vi "Should Show Spectrogram Window.vi"(11 "Data in":T1={"First Time"=FALSE, "Show Spectrogram Window"=TRUE, "Show Spectrogram Window Button Clicked"=FALSE, "Extension"=0, "Time steps"=-1, "Frequency bins"=512, "Type"=1, "Length"=-1, "Color Table"=0, "Spectrogram VI Ref"=refnum} {"Color Table" items=["Rainbow", "Inverse gray", "Gray", "Color table 1", "Color table 2", "Color table 3"]; "Type" items=["None ", "Hanning", "Hamming", "Blackman-Harris", "Exact Blackman", "Blackman", "Flat Top", "4 Term B-Harris ", "7 Term B-Harris", "Low Sidelobe", "Gaussian"]; "Extension" items=["Zero padding", "Symmetric", "Periodic"]}) -> (2 "Show Window":bool, 3 "Data out":T1={"First Time"=FALSE, "Show Spectrogram Window"=TRUE, "Show Spectrogram Window Button Clicked"=FALSE, "Extension"=0, "Time steps"=-1, "Frequency bins"=512, "Type"=1, "Length"=-1, "Color Table"=0, "Spectrogram VI Ref"=refnum} {"Color Table" items=["Rainbow", "Inverse gray", "Gray", "Color table 1", "Color table 2", "Color table 3"]; "Type" items=["None ", "Hanning", "Hamming", "Blackman-Harris", "Exact Blackman", "Blackman", "Flat Top", "4 Term B-Harris ", "7 Term B-Harris", "Low Sidelobe", "Gaussian"]; "Extension" items=["Zero padding", "Symmetric", "Periodic"]})   [LabVIEW 2023, in "Spectrogram.lvlib" / "Spectrogram.lvclass"]
uses:
  Spectrogram.lvclass
  Spectrogram Data.ctl
  Spectrogram.lvclass/Spectrogram.ctl
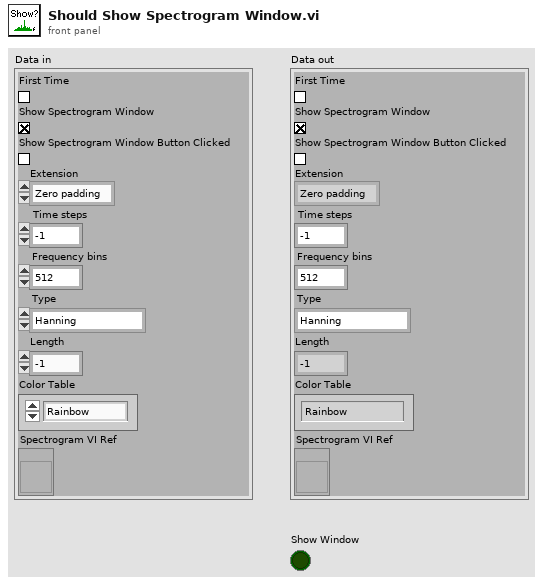
[diagram p1: front panel]
types:
  T1 = typedef "Spectrogram.lvlib/Spectrogram.lvclass/Spectrogram Data.ctl" = cluster{"First Time":bool, "Show Spectrogram Window":bool, "Show Spectrogram Window Button Clicked":bool, "Extension":u16, "Time steps":i32, "Frequency bins":i32, "Type":i32, "Length":i32, "Color Table":u16, "Spectrogram VI Ref":refnum<vi>}
  T2 = enum32{"Invalid", "Standard", "Closed", "Hidden", "Minimized", "Maximized"}
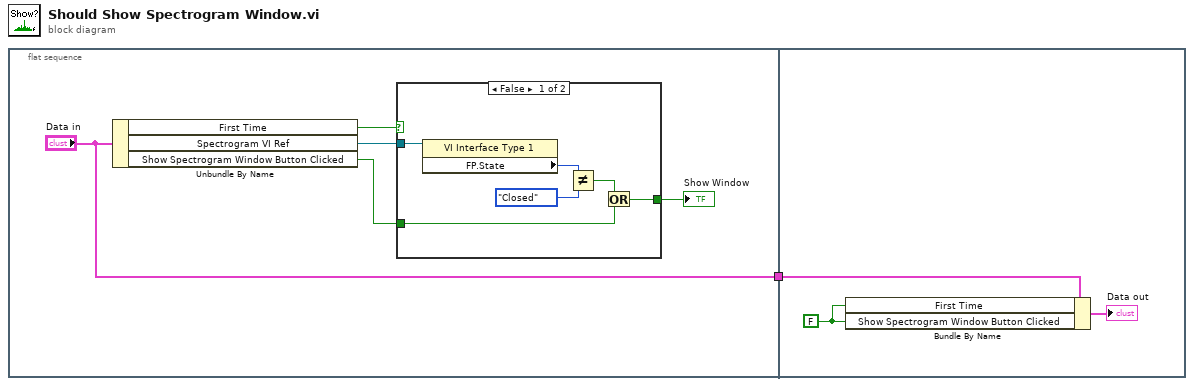
[diagram p0: block diagram]
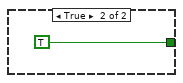
[diagram p2: hidden frame]
diagram:
  n1 = flat-sequence {
    tunnel: ["Data in"] -> w1
    tunnel: w1 -> [w16]
    frame #0 {
      n2 = Unbundle By Name("Data in") -> ("First Time"=w2:bool, "Spectrogram VI Ref"=w5:refnum<vi>, "Show Spectrogram Window Button Clicked"=w4:bool)
      n3 = case shown="False" w2 {
        tunnel: w5 -> [w12 _]
        tunnel: [w7 TRUE] -> w6
        tunnel: w4 -> [w9 _]
        frame False {
          n4 = property class="VI Interface Type 1"(reference=w12) -> ("FP.State"=w11:T2)  [unwired: 1 in, 2 out]
          n5 = Not Equal?(x=w11, y=T2."Closed" ("Front Panel Window:State")) -> (x != y?=w8:bool)
          n6 = Or(x=w8, y=w9) -> (x .or. y?=w7:bool)
        }
        frame True {
        }
      }
      "Show Window" <- w6
    }
    frame #1 {
      w14 = FALSE ("Show Spectrogram Window Button Clicked")
      n7 = Bundle By Name(cluster=w16, "First Time"=w14, "Show Spectrogram Window Button Clicked"=w14) -> (→"Data out":T1)
    }
  }
